vi "simpletls bench.vi"() -> ()   [LabVIEW 2016]
uses:
  lvlibtls/tls library paths.vi
  lvlibtls/lv tls dll.lvlib
panel:
  out "x/y 2":dbl format="%^#_11e"
  out "Numeric 2":u64
  out "Numeric":u64
  out "x-y":dbl
  in  "dimension size":i32=10000
  out "x/y":dbl format="%^#_11e"
  in  "stop":bool
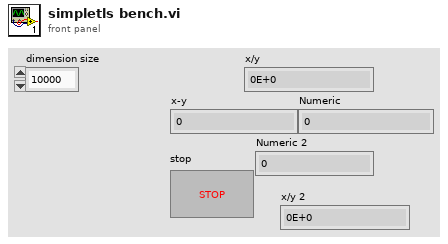
[diagram p1: front panel]
types:
  T1 = enum16{"Standard", "Buffered", "CRLF", "Immediate"}
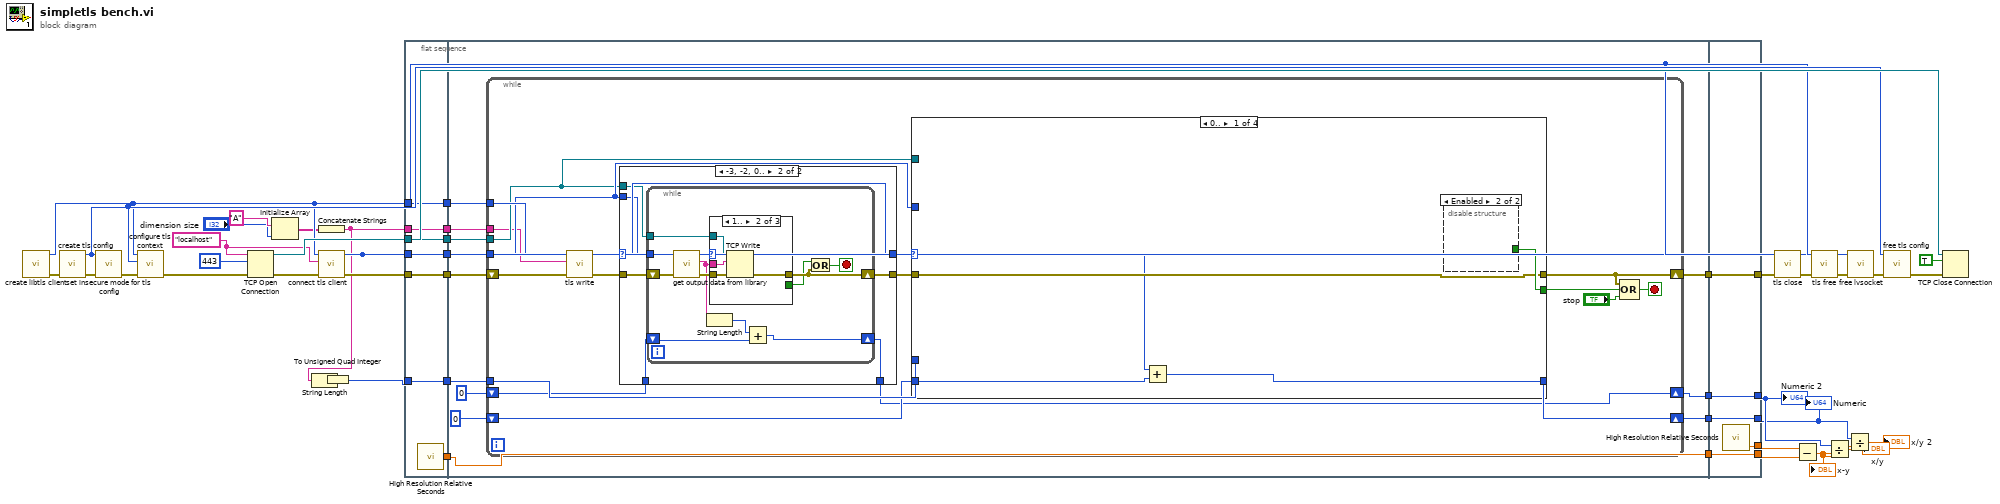
[diagram p0: block diagram]
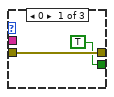
[diagram p3: hidden frame]
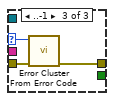
[diagram p4: hidden frame]
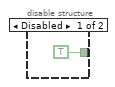
[diagram p5: hidden frame]
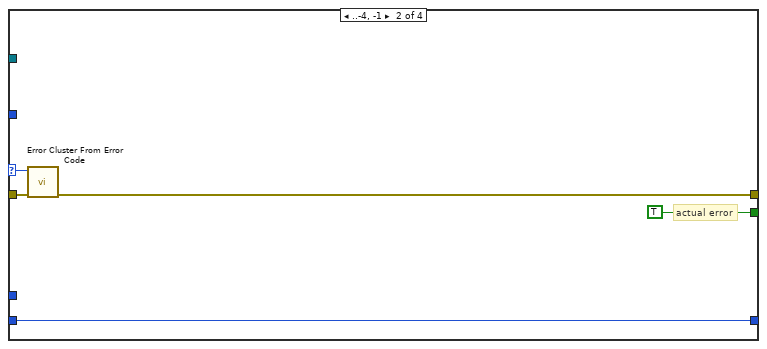
[diagram p6: hidden frame]
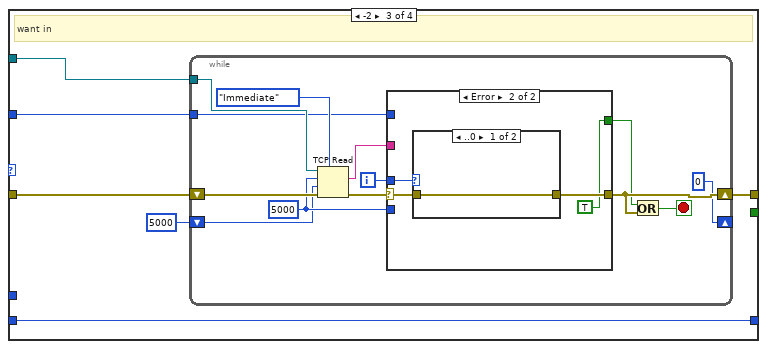
[diagram p7: hidden frame]
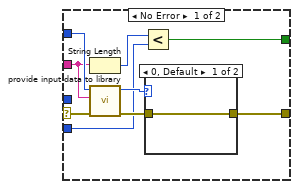
[diagram p8: hidden frame]
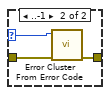
[diagram p9: hidden frame]
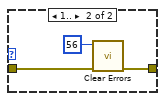
[diagram p10: hidden frame]
diagram:
  w35 = "localhost" ("address")
  n1 = call "create libtls client.vi"() -> ("error out"=w34:errorcluster, "client out"=w27:u64)  [unwired: 10 in]
  n2 = call "create tls config.vi"("error in"=w34) -> ("error out"=w33:errorcluster, "config out"=w32:u64)  [unwired: 9 in]
  n3 = call "set insecure mode for tls config.vi"("error in"=w33, "config in"=w32) -> ("error out"=w39:errorcluster)  [unwired: 9 in]
  n4 = call "configure tls context.vi"("error in"=w39, "config"=w32, "context"=w27) -> ("error out"=w38:errorcluster)  [unwired: 8 in]
  n5 = TCP Open Connection(address=w35, remote port or service name=u16 443, error in (no error)=w38) -> (connection ID=w40:refnum<k5>, error out=w37:errorcluster)  [unwired: 2 in]
  n6 = Initialize Array("A" ("address"), "dimension size") -> (w23:string[])
  n7 = Concatenate Strings(w23) -> (w11:string)
  n8 = String Length(string=w11) -> (length=w9:i32)
  n9 = call "connect tls client.vi"("error in"=w37, "servername"=w35, "client"=w27) -> ("error out"=w36:errorcluster, "lvsocket"=w26:u64)  [unwired: 7 in]
  n10 = To Unsigned Quad Integer(1:w9) -> (0:w6:u64)
  n11 = flat-sequence {
    tunnel: w11 -> [w45]
    tunnel: w26 -> [w46]
    tunnel: w27 -> [w47]
    tunnel: w36 -> [w48]
    tunnel: w40 -> [w49]
    tunnel: [w49] -> w21
    tunnel: [w48] -> w20
    tunnel: [w47] -> w19
    tunnel: [w46] -> w18
    tunnel: [w45] -> w17
    tunnel: [w44] -> w14
    tunnel: [w43] -> w10
    tunnel: w6 -> [w43]
    tunnel: w21 -> [w60]
    tunnel: w20 -> [w59]
    tunnel: w19 -> [w58]
    tunnel: w18 -> [w57]
    tunnel: w17 -> [w56]
    tunnel: [w61] -> w16
    tunnel: w14 -> [w55]
    tunnel: [w55] -> w13
    tunnel: w10 -> [w54]
    tunnel: [w52] -> w8
    tunnel: [w50] -> w5
    tunnel: [w168] -> w41
    tunnel: w16 -> [w168]
    tunnel: [w167] -> w15
    tunnel: w13 -> [w166]
    tunnel: [w166] -> w12
    tunnel: [w165] -> w2
    tunnel: w8 -> [w165]
    tunnel: [w164] -> w4
    tunnel: w5 -> [w164]
    frame #0 {
      n12 = call <vilib>:"High Resolution Relative Seconds.vi"() -> ("relative seconds"=w44:dbl)
    }
    frame #1 {
      n13 = while {
        shift-right: [w78] -> w61
        shift-left: w59 -> [w79]
        tunnel: w58 -> [w77]
        tunnel: w60 -> [w69]
        tunnel: w57 -> [w70]
        tunnel: w56 -> [w68]
        tunnel: w54 -> [w66]
        shift-right: [w65] -> w52
        shift-left: u64 0 -> [w64]
        shift-right: [w62] -> w50
        shift-left: u64 0 -> [w63]
        stop <- w76 stop-if-true
        n14 = call "tls write.vi"("error in"=w79, "data"=w68, "tls context"=w77) -> ("error out"=w71:errorcluster, "error response"=w74:i32)  [unwired: 7 in]
        n15 = case shown="-3, -2, 0.." w74 {
          selector: w74 -> [w81 w89]
          tunnel: [w81 w89] -> w73
          tunnel: [w82 w87] -> w72
          tunnel: w71 -> [w82 w88]
          tunnel: w70 -> [_ w86]
          tunnel: w69 -> [_ w85]
          tunnel: w63 -> [w80 w84]
          tunnel: [w80 w83] -> w62
          frame Default {
          }
          frame -3, -2, 0.. {
            n16 = while {
              shift-right: [w98] -> w87
              shift-left: w88 -> [w101]
              tunnel: w86 -> [w97]
              tunnel: w85 -> [w96]
              shift-right: [w90] -> w83
              shift-left: w84 -> [w91]
              stop <- w95 stop-if-true
              n17 = call "get output data from library.vi"("error in"=w101, "lvsocket"=w97) -> ("error out"=w100:errorcluster, "data"=w93:string, "err"=w99:i32)  [unwired: 7 in]
              n18 = String Length(string=w93) -> (length=w92:i32)
              n19 = case shown="1.." w99 {
                selector: w99 -> [_ _ w109]
                tunnel: w100 -> [w103 w107 w110]
                tunnel: [w103 w106 w108] -> w98
                tunnel: w93 -> [_ w105 _]
                tunnel: w96 -> [_ w104 _]
                tunnel: [TRUE _ _] -> w94
                frame 0 {
                }
                frame 1.. {
                  n20 = TCP Write(connection ID=w104, data in=w105, error in (no error)=w107) -> (error out=w106:errorcluster)  [unwired: 1 in, 2 out]
                }
                frame ..-1 {
                  n21 = call <vilib>:"Error Cluster From Error Code.vi"("error in (no error)"=w110, "error code (0)"=w109) -> ("error out"=w108:errorcluster)  [unwired: 7 in]
                }
              }
              n22 = Add(x=w92, y=w91) -> (x+y=w90:u64)
              n23 = Or(x=w94, y=w98) -> (x .or. y?=w95:bool)
            }
          }
        }
        n24 = case shown="0.." w73 {
          selector: w73 -> [w111 w121 _ _]
          tunnel: [w114 w120 w125 w163] -> w78
          tunnel: [w115 TRUE _ _] -> w75
          tunnel: w69 -> [_ _ w127 _]
          tunnel: w70 -> [_ _ w126 _]
          tunnel: w72 -> [w114 w118 w124 w163]
          tunnel: w66 -> [_ _ _ _]
          tunnel: [w113 w117 w122 w162] -> w65
          tunnel: w64 -> [w112 w117 w122 w162]
          frame 0.. {
            n25 = Add(x=w111, y=w112) -> (x+y=w113:u64)
            n26 = disable-structure shown="Enabled" {
              disable-tunnel: [TRUE _] -> w115
              frame Disabled {
              }
              frame Enabled {
              }
            }
          }
          frame ..-4, -1 {
            # "actual error"
            n27 = call <vilib>:"Error Cluster From Error Code.vi"("error in (no error)"=w118, "error code (0)"=w121) -> ("error out"=w120:errorcluster)  [unwired: 7 in]
          }
          frame -2 {
            # "want in"
            n28 = while {
              tunnel: w127 -> [w140]
              tunnel: w126 -> [w137]
              shift-right: [w135] -> w125
              shift-left: w124 -> [w136]
              shift-right: [0 ("timeout ms (25000)")] -> _
              shift-left: 5000 ("timeout ms (25000)") -> [w129]
              i -> [w134]
              stop <- w133 stop-if-true
              w131 = 5000 ("bytes to read")
              n29 = TCP Read(connection ID=w140, bytes to read=w131, error in (no error)=w136, 7:T1."Immediate" ("mode (standard)"), 9:w129) -> (data out=w130:string, error out=w138:errorcluster)  [unwired: 1 out]
              n30 = case shown="Error" w138 {
                selector: w138 -> [w149 w157]
                tunnel: w130 -> [w141 _]
                tunnel: w137 -> [w142 _]
                tunnel: [w146 w156] -> w135
                tunnel: w134 -> [_ w155]
                tunnel: [w143 TRUE] -> w132
                tunnel: w131 -> [w144 _]
                frame No Error {
                  n31 = String Length(string=w141) -> (length=w145:i32)
                  n32 = call "provide input data to library.vi"("error in"=w149, "data in"=w141, "lvsocket"=w142) -> ("error out"=w148:errorcluster, "return"=w147:i32)  [unwired: 7 in]
                  n33 = Less?(x=w145, y=w144) -> (x < y?=w143:bool)
                  n34 = case shown="0, Default" w147 {
                    selector: w147 -> [_ w152]
                    tunnel: w148 -> [w150 w153]
                    tunnel: [w150 w151] -> w146
                    frame 0, Default {
                    }
                    frame ..-1 {
                      n35 = call <vilib>:"Error Cluster From Error Code.vi"("error in (no error)"=w153, "error code (0)"=w152) -> ("error out"=w151:errorcluster)  [unwired: 7 in]
                    }
                  }
                }
                frame Error {
                  n36 = case shown="..0" w155 {
                    tunnel: w157 -> [w158 w161]
                    tunnel: [w158 w160] -> w156
                    frame ..0 {
                    }
                    frame 1.. {
                      n37 = call <vilib>:"Clear Errors.vi"("error in (no error)"=w161, "specific error code to clear (0: all)"=56) -> ("error out"=w160:errorcluster)  [unwired: 4 in, 1 out]
                    }
                  }
                }
              }
              n38 = Or(x=w132, y=w135) -> (x .or. y?=w133:bool)
            }
          }
          frame -3 {
            # "want out"
          }
        }
        n39 = Compound Arithmetic op=OR(w78, w75, "stop") -> (w76:bool)
      }
    }
    frame #2 {
      n40 = call <vilib>:"High Resolution Relative Seconds.vi"() -> ("relative seconds"=w167:dbl)
    }
  }
  n41 = call "tls close.vi"("error in"=w41, "tls context"=w27) -> ("error out"=w29:errorcluster)  [unwired: 8 in, 1 out]
  n42 = Subtract(x=w15, y=w12) -> (x-y=w1:dbl)
  "x-y" <- w1
  n43 = call "tls free.vi"("error in"=w29, "tls context"=w27) -> ("error out"=w30:errorcluster)  [unwired: 9 in]
  n44 = Divide(x=w4, y=w1) -> (x/y=→"x/y":dbl)
  n45 = Divide(x=w2, y=w1) -> (x/y=→"x/y 2":dbl)
  n46 = call "free lvsocket.vi"("error in"=w30, "lvsocket"=w26) -> ("error out"=w28:errorcluster)  [unwired: 9 in]
  n47 = call "free tls config.vi"("error in"=w28, "config"=w32) -> ("error out"=w31:errorcluster)  [unwired: 9 in]
  n48 = TCP Close Connection(connection ID=w40, abort (F)=TRUE, error in (no error)=w31) -> ()  [unwired: 2 out]
  "Numeric" <- w2
  "Numeric 2" <- w4
